vi "setup.vi"(0 "para0":string, 1 "para1":string, 2 "para2":string, 3 "para3":string, 4 "para4":string, 5 "para5":string, 6 "para6":string, 7 "error in (no error)":errorcluster caption="entrée d'erreur (pas d'erreur)") -> (18 "function return":i32, 20 "para0 out":string, 21 "para1 out":string, 22 "para2 out":string, 23 "para3 out":string, 24 "para4 out":string, 25 "para5 out":string, 26 "para6 out":string, 27 "error out":errorcluster caption="sortie d'erreur")   [LabVIEW 2020, in "Library Instrument & Equipement.lvlib" / "Library Printer.lvlib" / "TSCLIB.lvlib"]
doc: "EXPORT int CALLBACK setup (char *,char *,char *,char *,char *,char *,char *);"
uses:
  TSCLIB.lvlib
  TSCLIB.dll
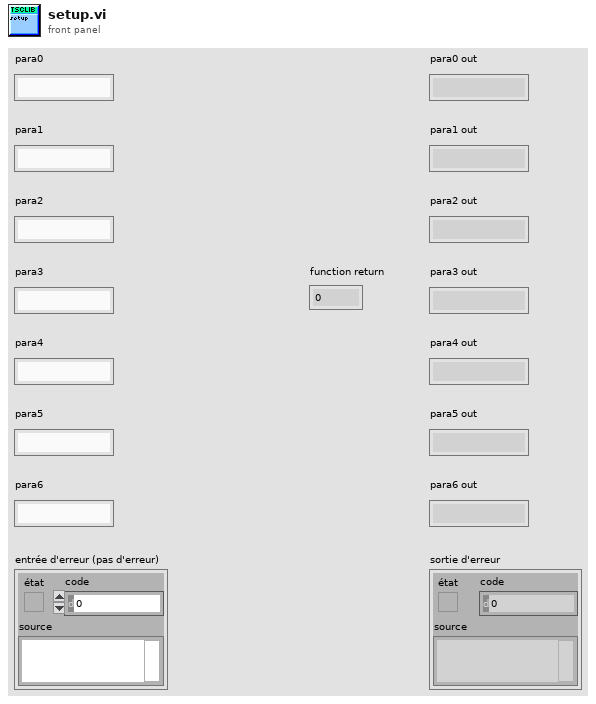
[diagram p1: front panel]
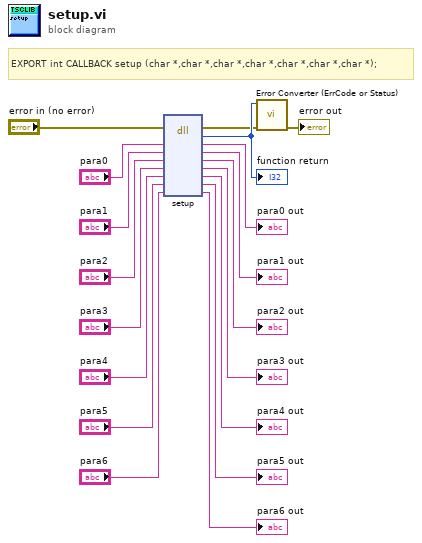
[diagram p0: block diagram]
diagram:
  # "EXPORT int CALLBACK setup (char *,char *,char *,char *,char *,char *,char *);"
  n1 = dll-call lib="C:/Users/ngarcin/OneDrive - Altyor/Standard TB/Class/Printer/Printer TSC/TSCLIB/TSCLIB.*" fn="setup"(error in="error in (no error)", "para0"="para0", "para1"="para1", "para2"="para2", "para3"="para3", "para4"="para4", "para5"="para5", "para6"="para6") -> (error out=w2:errorcluster, w18:i32, "para0"=→"para0 out":string, "para1"=→"para1 out":string, "para2"=→"para2 out":string, "para3"=→"para3 out":string, "para4"=→"para4 out":string, "para5"=→"para5 out":string, "para6"=→"para6 out":string)  [unwired: 2 in, 1 out]
  "function return" <- w18
  n2 = call "Error Converter (ErrCode or Status).vi"("error in (no error)"=w2, "error code"=w18) -> ("error out"=→"error out":errorcluster)  [unwired: 9 in]
